vi "Tell Child Forward.vi"(4 "Alias":string, 6 "Msg":refnum<class "Msg.lvclass">, 7 "Actor in":refnum<class "Actor.lvclass">, 9 "Msg Attributes":T1 {"Teller"."Absolute Time" format="%<%x %.3X>T"}, 10 "Previous Told":bool) -> (0 "Error out":errorcluster, 1 "Told":bool, 2 "Told Or Previous Told":bool, 5 "Actor out":refnum<class "Actor.lvclass">)   [LabVIEW 2020, in "jettl.lvlib"]
uses:
  jettl.lvlib
  Actor/Actor.lvclass
  Relation.ctl
  Msg/Msg.lvclass
  Teller.ctl
  Msg Input/Msg Input.lvclass
  Msg Output/Msg Output.lvclass
  Msg Attributes.ctl
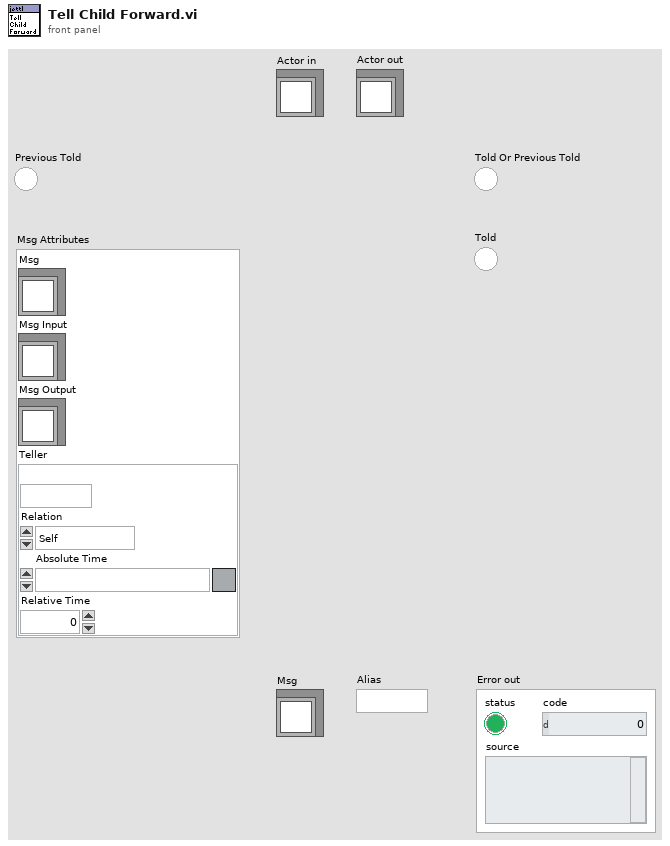
[diagram p1: front panel]
types:
  T1 = typedef "jettl.lvlib/Msg Attributes.ctl" = cluster{"Msg":refnum<class "Msg.lvclass">, "Msg Input":refnum<class "Msg Input.lvclass">, "Msg Output":refnum<class "Msg Output.lvclass">, "Teller":T2}
  T2 = typedef "jettl.lvlib/Teller.ctl" = cluster{"Alias":string, "Relation":T3, "Absolute Time":timestamp, "Relative Time":dbl}
  T3 = typedef "jettl.lvlib/Relation.ctl" = enum16{"Self", "Parent", "Child"}
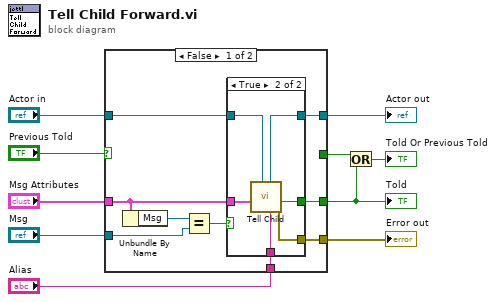
[diagram p0: block diagram]
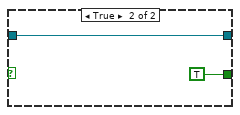
[diagram p3: hidden frame]
diagram:
  n1 = case shown="False" "Previous Told" {
    tunnel: "Actor in" -> [w19 w28]
    tunnel: [w18 _] -> w9
    tunnel: [w17 w28] -> w8
    tunnel: "Msg Attributes" -> [w13 _]
    tunnel: "Msg" -> [w12 _]
    tunnel: [w16 _] -> w1
    tunnel: "Alias" -> [w15 _]
    tunnel: [_ TRUE ("Told Or Previous Told")] -> w3
    frame False {
      n2 = Unbundle By Name(w13) -> ("Msg"=w14:refnum<class "Msg.lvclass">)
      n3 = Equal?(x=w14, y=w12) -> (x = y?=w11:bool)
      n4 = case shown="True" w11 {
        tunnel: w19 -> [w20 w26]
        tunnel: [_ w24] -> w18
        tunnel: [w20 w25] -> w17
        tunnel: w13 -> [_ w21]
        tunnel: [_ w23] -> w16
        tunnel: w15 -> [_ w22]
        frame False {
        }
        frame True {
          n5 = call "Tell Child.vi"("Alias"=w22, "Actor in"=w26, "Msg Attributes"=w21) -> ("Error out"=w24:errorcluster, "Told"=w23:bool, "Actor out"=w25:refnum<class "Actor.lvclass">)  [unwired: 6 in]
        }
      }
    }
    frame True {
    }
  }
  "Error out" <- w9
  "Actor out" <- w8
  "Told" <- w1
  n6 = Or(x=w3, y=w1) -> (x .or. y?=→"Told Or Previous Told":bool)
